vi "scan.vi"(8 "error in (no error)":errorcluster, 11 "Input":string="0,-110n,10n,64") -> (0 "error out":errorcluster, 3 "Output":string)   [LabVIEW 2014]
uses:
  <userlib>/Nanonis Prog Interface V5/Nanonis Prog Interface.lvlib
panel:
  in  "seconds to wait":dbl=3.0
  in  "Angle (deg)":sgl=nan caption="Angle (deg) (NaN=no change)" format="%.2f"
  in  "Size (m)":cluster{"Width":sgl, "Height":sgl}={"Width"=1e-08, "Height"=1e-08} caption="Size (m) (NaN=no change)" {"Height" format="%.2p"; "Width" format="%.2p"}
  out "size(s)":i32=4
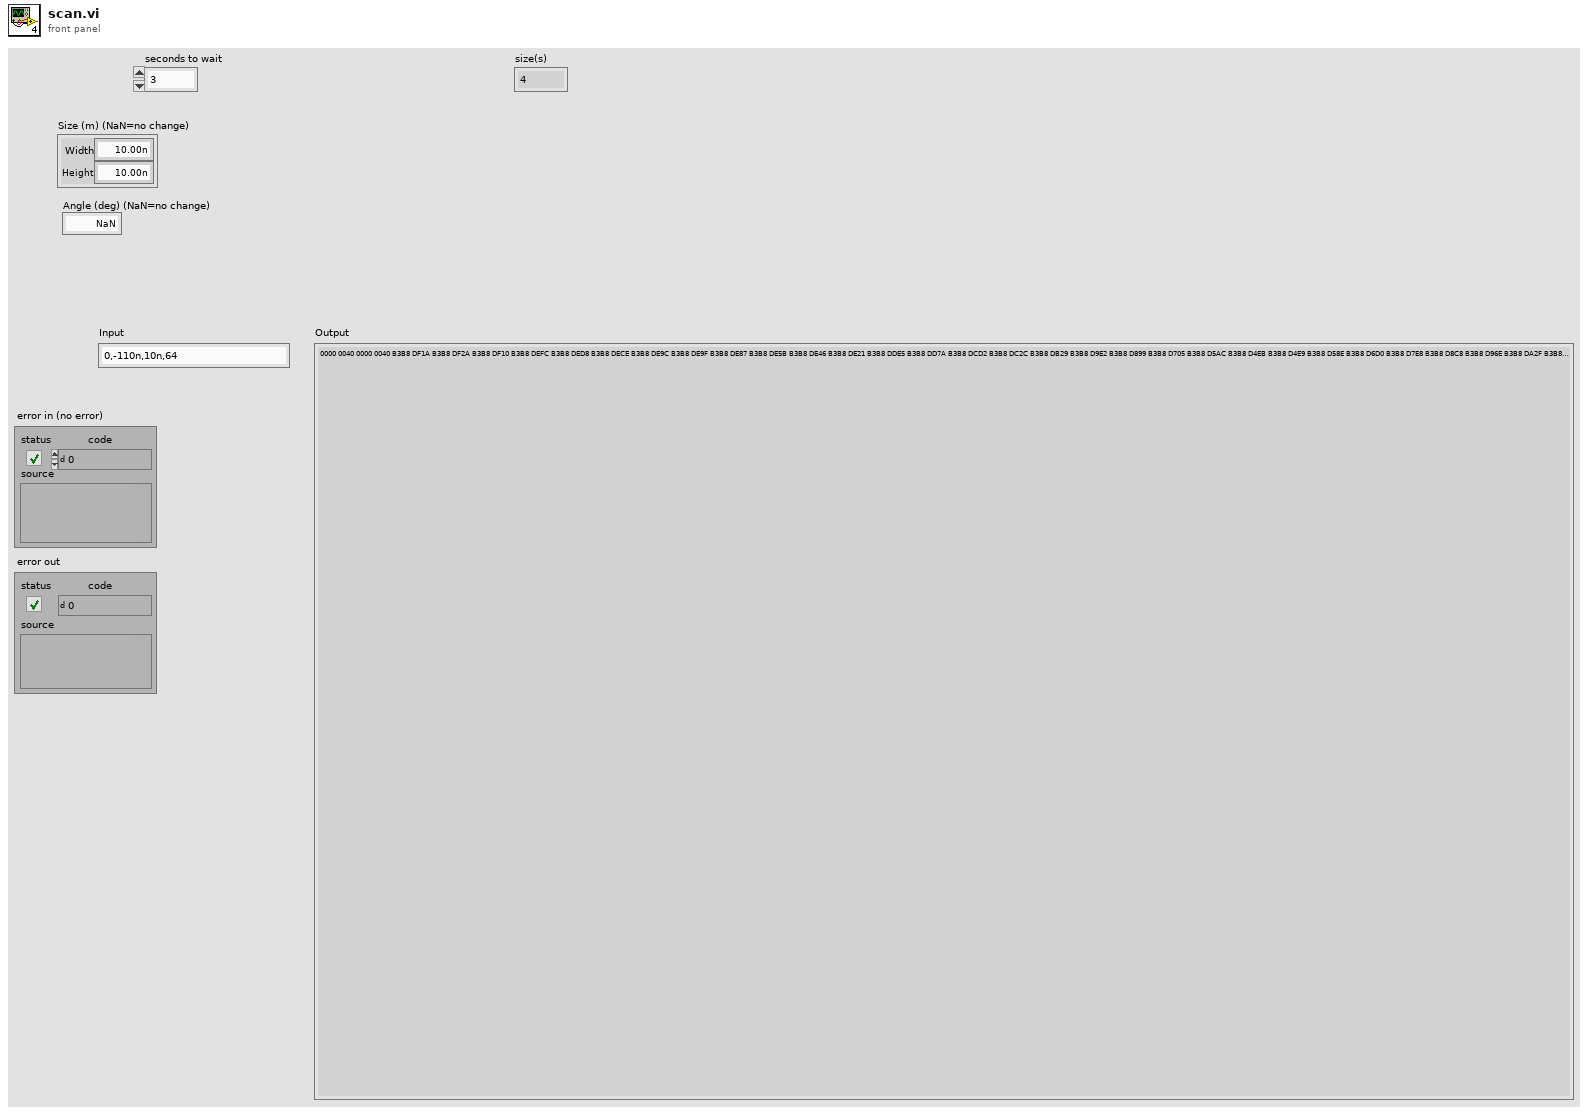
[diagram p1: front panel]
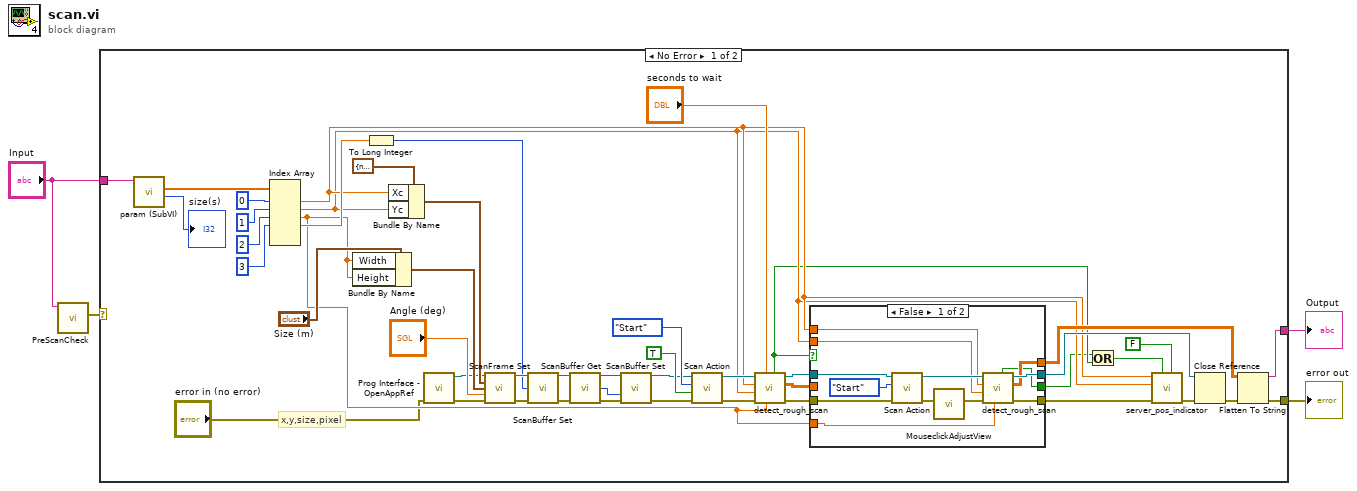
[diagram p0: block diagram]
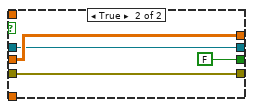
[diagram p2: hidden frame]
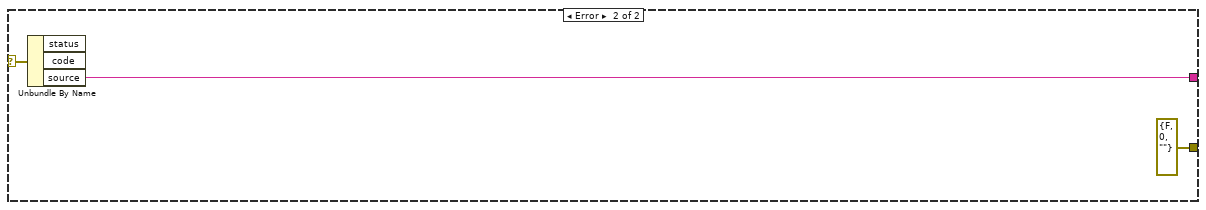
[diagram p3: hidden frame]
diagram:
  n1 = call "PreScanCheck.vi"("Input"="Input") -> ("error"=w1:errorcluster)  [unwired: 8 in, 2 out]
  n2 = case shown="No Error" w1 {
    selector: w1 -> [_ w71]
    tunnel: [w35 w70] -> w4
    tunnel: [w27 errorcluster {"status"=FALSE, "code"=0, "source"=""} ("error out")] -> w3
    tunnel: "Input" -> [w23 _]
    frame No Error {
      # "x,y,size,pixel"
      n3 = call <userlib>:"param (SubVI).vi"("Input"=w23) -> ("num"=→"size(s)":i32, "parm"=w51:dbl[])  [unwired: 8 in, 1 out]
      n4 = Index Array(array=w51, index #1=0 ("index"), index #2=1 ("index"), index #3=2 ("index"), index #4=3 ("index")) -> (element #1=w15:dbl, element #2=w14:dbl, element #3=w13:dbl, element #4=w37:dbl)  [unwired: 2 in, 2 out]
      n5 = Bundle By Name(cluster="Size (m)", "Width"=w13, "Height"=w13) -> (w38:cluster{"Width":sgl, "Height":sgl})
      n6 = To Long Integer(number=w37) -> (32bit integer=w36:i32)
      n7 = Bundle By Name(cluster=cluster{"Xc":sgl, "Yc":sgl} {"Xc"=nan, "Yc"=nan} ("Center coordinates (m)"), "Xc"=w15, "Yc"=w14) -> (w49:cluster{"Xc":sgl, "Yc":sgl})
      n8 = call <userlib>:"Prog Interface - OpenAppRef.vi"("Error in (no error)"="error in (no error)") -> ("Error out"=w12:errorcluster, "Application reference"=w24:refnum<vi>)  [unwired: 5 in]
      n9 = call <userlib>:"ScanFrame Set.vi"("Application ref in"=w24, "Center coordinates (m)"=w49, "Size (m)"=w38, "Angle (deg)"="Angle (deg)", "error in (no error)"=w12) -> ("Application ref out"=w47:refnum<vi>, "error out"=w46:errorcluster)  [unwired: 9 in]
      n10 = call <userlib>:"ScanBuffer Set.vi"("Application ref in"=w47, "Pixels"=w36, "error in (no error)"=w46) -> ("Application ref out"=w31:refnum<vi>, "error out"=w30:errorcluster)  [unwired: 11 in]
      n11 = call <userlib>:"ScanBuffer Get.vi"("Application ref in"=w31, "error in (no error)"=w30) -> ("Application ref out"=w33:refnum<vi>, "Pixels/line"=w34:i32, "error out"=w32:errorcluster)  [unwired: 9 in, 2 out]
      n12 = call <userlib>:"ScanBuffer Set.vi"("Application ref in"=w33, "Lines"=w34, "error in (no error)"=w32) -> ("Application ref out"=w29:refnum<vi>, "error out"=w28:errorcluster)  [unwired: 11 in]
      n13 = call <userlib>:"Scan Action.vi"("error in (no error)"=w28, "Direction: up/down (T=up)"=TRUE, "Scan action (Start)"=enum16{"Start", "Stop", "Pause", "Resume"}."Start", "Application ref in"=w29) -> ("error out"=w18:errorcluster, "Application ref out"=w19:refnum<vi>)  [unwired: 5 in]
      n14 = call "detect_rough_scan.vi"("size (m)"=w13, "max scan time"="seconds to wait", "Error in"=w18, "Y (m)"=w14, "X (m)"=w15, "App in"=w19) -> ("error out"=w10:errorcluster, "Array"=w16:sgl[][], "Application ref out"=w17:refnum<vi>, "rough image detected"=w6:bool)  [unwired: 2 in]
      n15 = case shown="False" w6 {
        tunnel: [w65 w68] -> w22
        tunnel: [w64 w67] -> w9
        tunnel: [w61 w69] -> w21
        tunnel: w17 -> [w58 w68]
        tunnel: w10 -> [w57 w67]
        tunnel: w16 -> [_ w69]
        tunnel: w15 -> [w56 _]
        tunnel: w14 -> [w55 _]
        tunnel: w13 -> [w54 _]
        tunnel: [w53 FALSE ("rough image detected")] -> w5
        frame False {
          n16 = call <userlib>:"Scan Action.vi"("error in (no error)"=w57, "Scan action (Start)"=enum16{"Start", "Stop", "Pause", "Resume"}."Start", "Application ref in"=w58) -> ("error out"=w59:errorcluster, "Application ref out"=w63:refnum<vi>)  [unwired: 6 in]
          n17 = call "MouseclickAdjustView.vi"("error in (no error)"=w59) -> ("error out"=w62:errorcluster)  [unwired: 10 in]
          n18 = call "detect_rough_scan.vi"("size (m)"=w54, "Error in"=w62, "Y (m)"=w55, "X (m)"=w56, "App in"=w63) -> ("error out"=w64:errorcluster, "Array"=w61:sgl[][], "Application ref out"=w65:refnum<vi>, "rough image detected"=w53:bool)  [unwired: 3 in]
        }
        frame True {
        }
      }
      n19 = Or(x=w5, y=w6) -> (x .or. y?=w7:bool)
      n20 = call "server_pos_indicator.vi"("reset"=FALSE, "rough"=w7, "error in"=w9, "yc"=w14, "xc"=w15) -> ("error out"=w8:errorcluster)  [unwired: 6 in]
      n21 = Close Reference(reference=w22, error in (no error)=w8) -> (error out=w25:errorcluster)
      n22 = Flatten To String(anything=w21, error in (no error)=w25) -> (data string=w35:string, error out=w27:errorcluster)  [unwired: 2 in, 1 out]
    }
    frame Error {
      n23 = Unbundle By Name(w71) -> ("source"=w70:string)  [unwired: 2 out]
    }
  }
  "Output" <- w4
  "error out" <- w3
